vi "IsDeviceReady.vi"(8 "error in (no error)":errorcluster, 11 "Camera_Prime95B in":refnum<class "Camera_Prime95B.lvclass">) -> (0 "error out":errorcluster, 2 "Ready?":bool, 3 "Camera_Prime95B out":refnum<class "Camera_Prime95B.lvclass">)   [LabVIEW 2020, in "Camera_Prime95B.lvlib" / "Camera_Prime95B.lvclass"]
uses:
  Camera_Prime95B.lvclass
  Camera_Prime95B.lvclass/Camera_Prime95B.ctl
  E:/Development/DevHardSoftware/MMicroscopyAF/Model/Real Hardware/Camera_Prime95B/Camera_Prime95B/Dependencies/PVCamNET.dll
  Dependencies/PVCamNET.dll
  HAL Layer/Component/Camera/Camera/Camera.lvclass
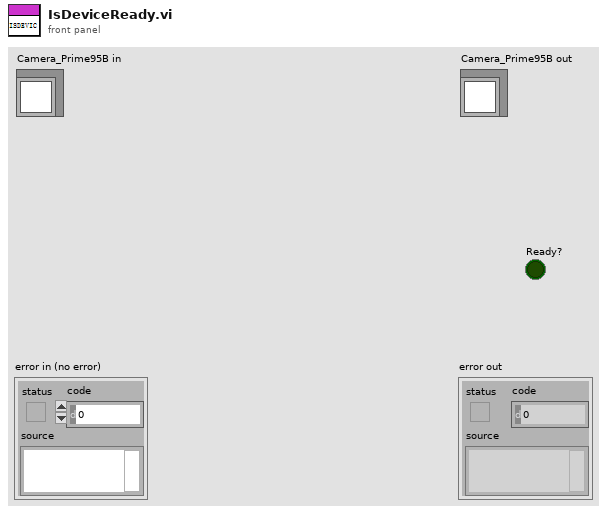
[diagram p1: front panel]
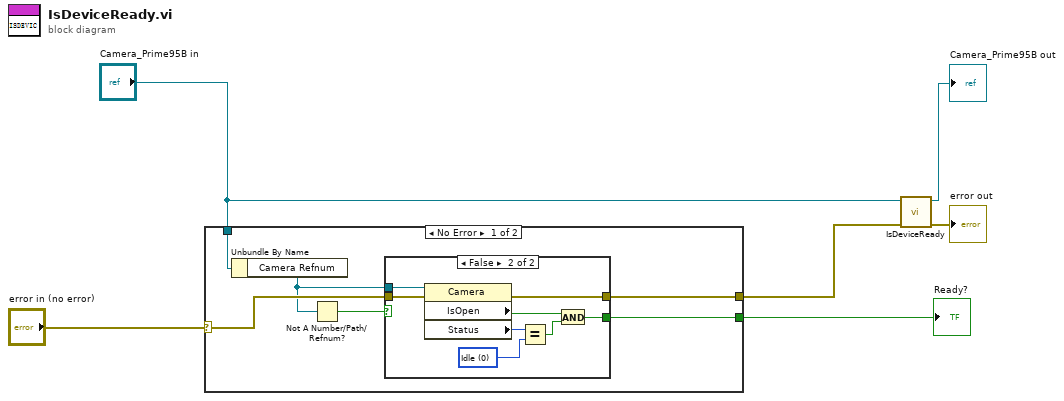
[diagram p0: block diagram]
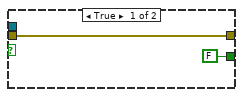
[diagram p2: hidden frame]
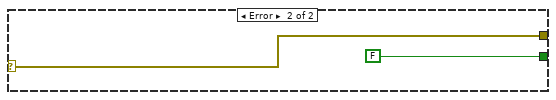
[diagram p3: hidden frame]
diagram:
  n1 = case shown="No Error" "error in (no error)" {
    selector: "error in (no error)" -> [w10 w24]
    tunnel: [w11 w24] -> w2
    tunnel: "Camera_Prime95B in" -> [w12 _]
    tunnel: [w7 FALSE] -> w1
    frame No Error {
      n2 = Unbundle By Name(w12) -> ("Camera Refnum"=w9:refnum<k24>)
      n3 = Not A Number/Path/Refnum?(number/path/refnum=w9) -> (NaN/Path/Refnum?=w8:bool)
      n4 = case shown="False" w8 {
        tunnel: w9 -> [_ w18]
        tunnel: [FALSE w17] -> w7
        tunnel: [w14 w16] -> w11
        tunnel: w10 -> [w14 w15]
        frame True {
        }
        frame False {
          w19 = 0 items=["Idle", "Capturing"] ("Status")
          n5 = property class="Camera"(reference=w18, error in=w15) -> (error out=w16:errorcluster, "IsOpen"=w21:bool, "Status"=w20:i32)  [unwired: 1 out]
          n6 = Equal?(x=w20, y=w19) -> (x = y?=w22:bool)
          n7 = And(x=w21, y=w22) -> (x .and. y?=w17:bool)
        }
      }
    }
    frame Error {
    }
  }
  "Ready?" <- w1
  n8 = call-parent "IsDeviceReady.vi"("error in (no error)"=w2, "Device in"="Camera_Prime95B in") -> ("error out"=→"error out":errorcluster, "Device out"=→"Camera_Prime95B out":refnum<class "Camera_Prime95B.lvclass">)  [unwired: 7 in, 1 out]
